vi "_GroupKill.vi"(1 "error in":errorcluster, 2 "group id":i32) -> (0 "error out":errorcluster)   [LabVIEW 2014, in "tango.lvlib"]
uses:
  tango.lvlib
  tango_binding.so
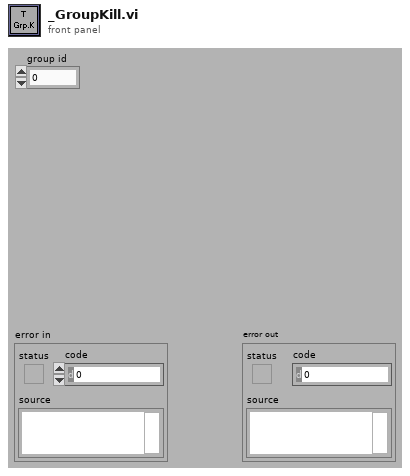
[diagram p1: front panel]
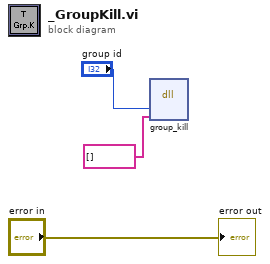
[diagram p0: block diagram]
diagram:
  n1 = dll-call lib="tango_binding.*" fn="group_kill"("group_id"="group id", "error_stack"=string[] [] ("error stack")) -> ()  [unwired: 6 in, 2 out]
  "error out" <- "error in"
